vi "Special_Project.vi"() -> ()   [LabVIEW 2025]
uses:
  <vilib>/Analysis/3filter.llb/Filter Passband Type.ctl
  <vilib>/Analysis/baseanly.llb/Mean (DBL).vi
  <vilib>/Analysis/3filter.llb/Butterworth Filter (DBL).vi
  <vilib>/Analysis/NI_AAL_SigProc.lvlib
  <vilib>/Analysis/NI_AALPro.lvlib
  <vilib>/Analysis/NI_AALBase.lvlib
panel:
  out "Max Baseline Shift Magnitude":dbl
  out "Baseline Shift Indicator":bool
  out "fs":dbl=360.0
  out "variability":dbl
  in  "file path":path
  out "# found 2":i32
  out "# found":i32
  out "DWT Reconstructed ECG":waveform(dbl)(graph)
  in  "noise amp":dbl=0.2 step=0.1
  out "Noisy ECG":dbl[](graph)
  in  "noise type":T1(ring)
  out "Raw ECG":dbl[](graph)
  in  "Duration (s)":dbl
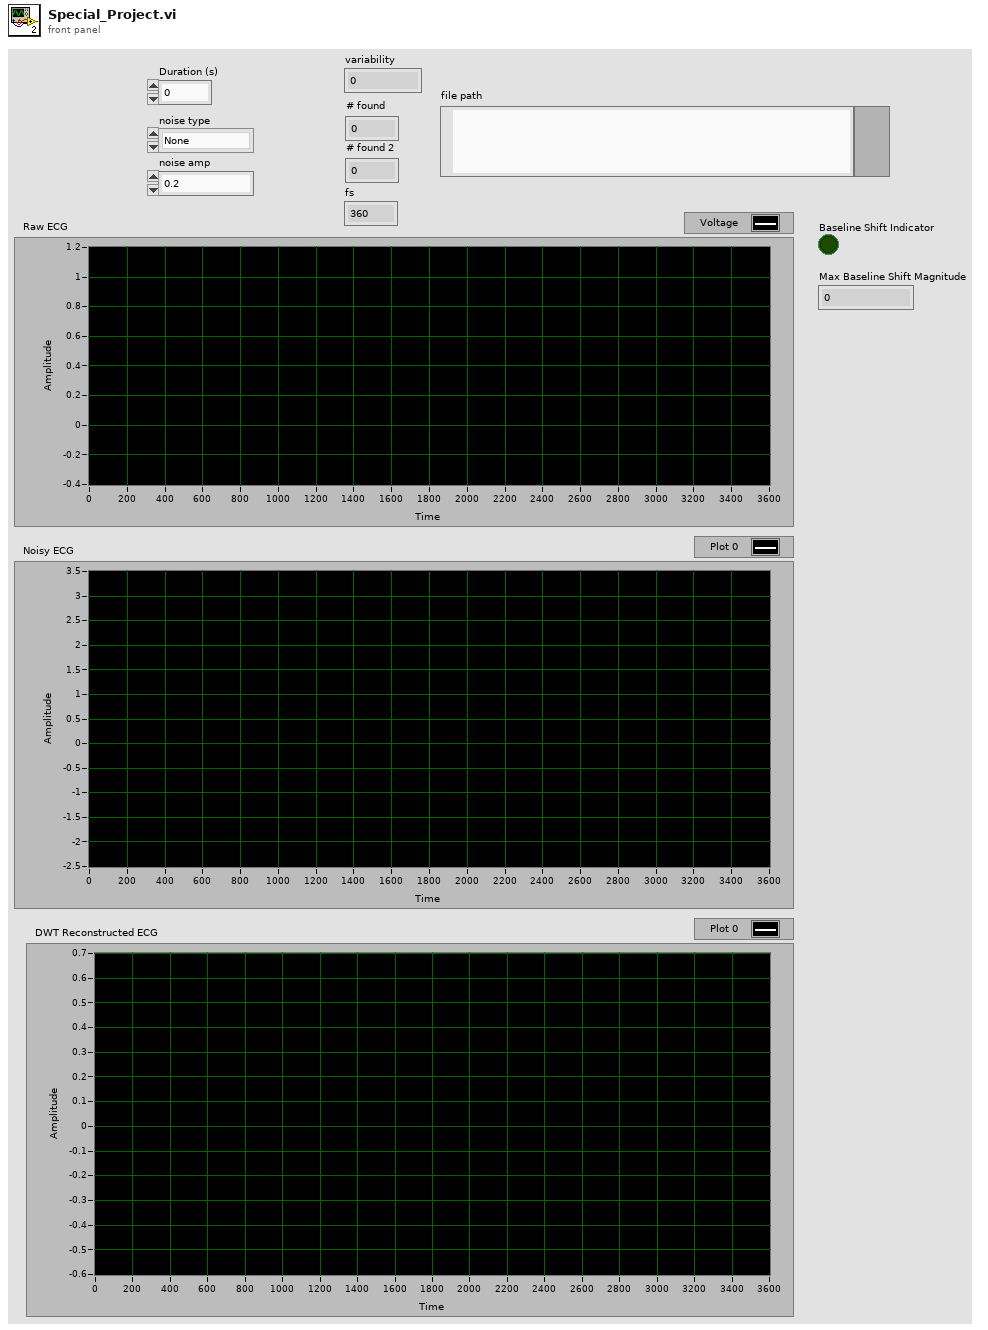
[diagram p1: front panel]
types:
  T1 = enum16{"None", "Slow Drift", "White noise", "Muscle artifact", "Motion artifact", "60 Hz"}
  T2 = typedef "NI_AALBase.lvlib/Filter Passband Type.ctl" = enum32{"Lowpass", "Highpass", "Bandpass", "Bandstop"}
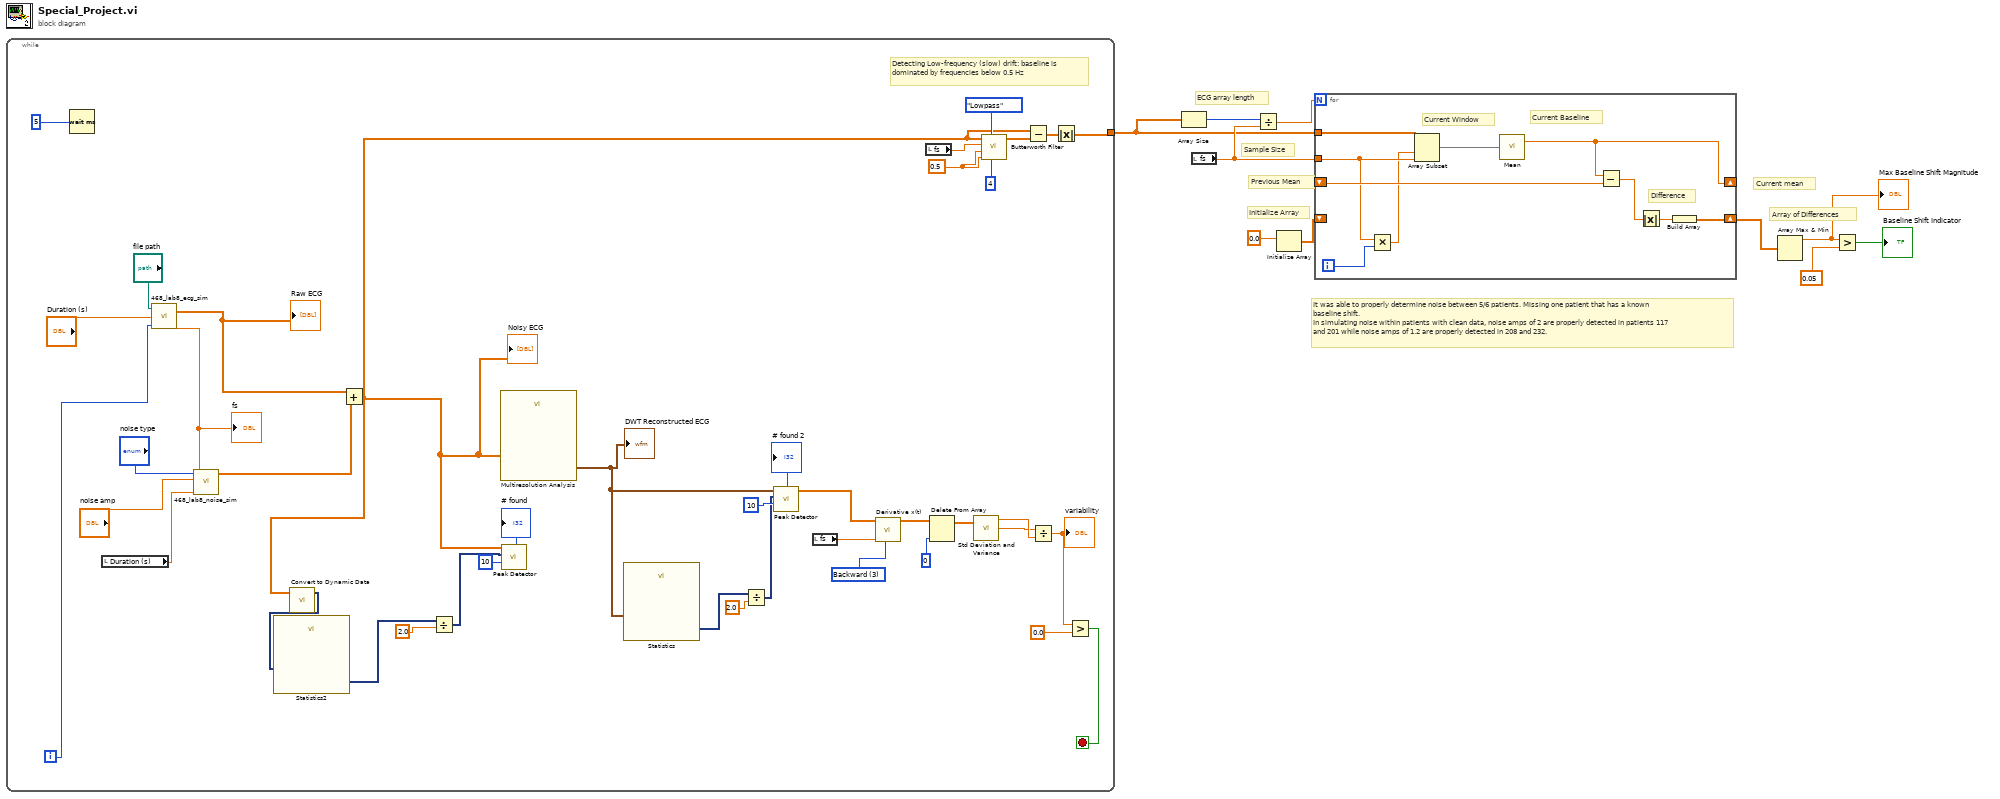
[diagram p0: block diagram]
diagram:
  # "Array of Differences"
  # "Initialize Array"
  # "Previous Mean"
  # "Current mean"
  # "Sample Size"
  # "ECG array length"
  # "It was able to properly determine noise between 5/6 patients. Missing one patient that has a known baseline shift. \nIn simulating noise within patients with clean data, noise amps of 2 are properly detected in patients 117 and 201 while noise amps of 1.2 are properly detected in 208 and 232."
  n1 = while {
    tunnel: [w14] -> w4
    i -> [w39]
    stop <- w11 stop-if-true
    w16 = 0.5 ("low cutoff freq: fl")
    w31 = u16 3 items=["2nd Order Central", "4th Order Central", "Forward", "Backward"] ("method")
    # "Detecting Low-frequency (slow) drift: baseline is dominated by frequencies below 0.5 Hz"
    n2 = Wait (ms)(milliseconds to wait=u32 5) -> ()  [unwired: 1 out]
    n3 = local read "Duration (s)"() -> (w33:dbl)
    n4 = call "468_lab8_ecg_sim.vi"("i"=w39, "duration"="Duration (s)", "file path"="file path") -> ("fs"=w36:dbl, "signal"=w23:dbl[])  [unwired: 1 in]
    "Raw ECG" <- w23
    "fs" <- w36
    n5 = call "468_lab8_noise_sim.vi"("duration"=w33, "fs"=w36, "noise amp"="noise amp", "noise type"="noise type") -> ("noise"=w37:dbl[])  [unwired: 3 in]
    n6 = Add(x=w23, y=w37) -> (x+y=w17:dbl[])
    "Noisy ECG" <- w17
    n7 = call "Convert to Dynamic Data"("Array"=w17) -> ("Dynamic Data Type"=w49:dynamicdata)  [unwired: 3 in]
    n8 = call "Statistics2"("Signals"=w49) -> ("Maximum"=w47:dynamicdata)  [unwired: 25 in, 1 out]
    n9 = Divide(x=w47, y=2.0) -> (x/y=w45:dynamicdata)
    n10 = call "Multiresolution Analysis"("Signal"=w17) -> ("Reconstruction"=w48:waveform(dbl))  [unwired: 9 in, 1 out]
    "DWT Reconstructed ECG" <- w48
    n11 = call <vilib>:"Peak Detector.vi"("width"=10, "threshold"=w45, "X"=w17) -> ("# found"=→"# found":i32)  [unwired: 4 in, 4 out]
    n12 = call "Statistics"("Signals"=w48) -> ("Maximum"=w43:dynamicdata)  [unwired: 25 in, 1 out]
    n13 = Divide(x=w43, y=2.0) -> (x/y=w41:dynamicdata)
    n14 = call <vilib>:"Peak Detector.vi"("width"=10, "threshold"=w41, "X"=w48) -> ("Locations"=w32:dbl[], "# found"=→"# found 2":i32)  [unwired: 4 in, 3 out]
    n15 = local read "fs"() -> (w25:dbl)
    n16 = call <vilib>:"Derivative x(t).vi"("method"=w31, "dt"=w25, "X"=w32) -> ("dX/dt"=w30:dbl[])  [unwired: 7 in, 1 out]
    n17 = local read "fs"() -> (w18:dbl)
    n18 = Delete From Array(array=w30, index=0) -> (array with subset deleted=w28:dbl[])  [unwired: 1 in, 1 out]
    n19 = call <vilib>:"Std Deviation and Variance.vi"("X"=w28) -> ("mean"=w27:dbl, "standard deviation"=w26:dbl)  [unwired: 1 in, 1 out]
    n20 = call-poly <vilib>:"Butterworth Filter.vi"("order"=4, "filter type"=Filter_Passband_Type."Lowpass", "low cutoff freq: fl"=w16, "high cutoff freq: fh"=w16, "sampling freq: fs"=w18, "X"=w17) -> ("Filtered X"=w20:dbl[])  [unwired: 2 in, 1 out]
    n21 = Subtract(x=w17, y=w20) -> (x-y=w19:dbl[])
    n22 = Divide(x=w26, y=w27) -> (x/y=w12:dbl)
    "variability" <- w12
    n23 = Absolute Value(x=w19) -> (abs(x)=w14:dbl[])
    n24 = Greater?(x=w12, y=0.0) -> (0:w11:bool)
  }
  n25 = Array Size(array=w4) -> (size(s)=w7:i32)
  n26 = local read "fs"() -> (w8:dbl)
  n27 = Divide(x=w7, y=w8) -> (x/y=w5:dbl)
  n28 = Initialize Array(0.0 ("element")) -> (w9:dbl[])  [unwired: 1 in]
  n29 = for {
    N: w5 -> [_]
    tunnel: w8 -> [w55]
    shift-right: [w61] -> _
    shift-left: _ -> [w60]
    shift-right: [w57] -> w10
    shift-left: w9 -> [_]
    tunnel: w4 -> [w53]
    i -> [w56]
    # "Difference"
    # "Current Baseline"
    # "Current Window"
    n30 = Multiply(x=w55, y=w56) -> (x*y=w54:dbl)
    n31 = Array Subset(array=w53, index=w54, length=w55) -> (w52:dbl[])
    n32 = call-poly <vilib>:"Mean.vi"("X"=w52) -> ("mean"=w61:dbl)  [unwired: 1 out]
    n33 = Subtract(x=w61, y=w60) -> (x-y=w59:dbl)
    n34 = Absolute Value(x=w59) -> (abs(x)=w58:dbl)
    n35 = Build Array(w58) -> (w57:dbl[])
  }
  n36 = Array Max & Min(array=w10) -> (max value=w1:dbl)  [unwired: 3 out]
  "Max Baseline Shift Magnitude" <- w1
  n37 = Greater?(x=w1, y=0.05) -> (0:→"Baseline Shift Indicator":bool)
